vi "format file size and count.vi"(11 "size":i64) -> (3 "size":string)   [LabVIEW 2023]
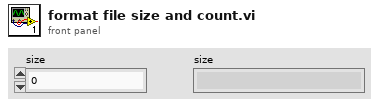
[diagram p1: front panel]
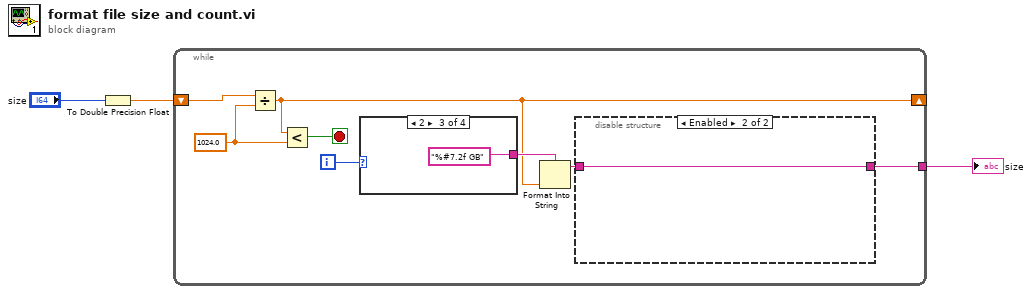
[diagram p0: block diagram]
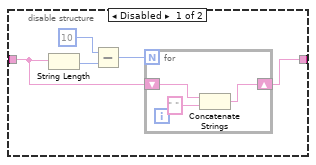
[diagram p2: hidden frame]
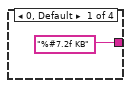
[diagram p3: hidden frame]
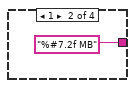
[diagram p4: hidden frame]
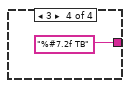
[diagram p5: hidden frame]
diagram:
  n1 = To Double Precision Float(number="size") -> (double precision float=w2:dbl)
  n2 = while {
    shift-right: [w6] -> _
    shift-left: w2 -> [w8]
    tunnel: [w4] -> w1
    i -> [w9]
    stop <- w10 stop-if-true
    w11 = 1024.0 ("y")
    n3 = Divide(x=w8, y=w11) -> (x/y=w6:dbl)
    n4 = Less?(x=w6, y=w11) -> (x < y?=w10:bool)
    n5 = case shown="2" w9 {
      tunnel: ["%#7.2f KB" ("String 2") "%#7.2f MB" ("String 2") "%#7.2f GB" ("String 2") "%#7.2f TB" ("String 2")] -> w7
      frame 0, Default {
      }
      frame 1 {
      }
      frame 2 {
      }
      frame 3 {
      }
    }
    n6 = Format Into String(format string=w7, w6) -> (resulting string=w5:string)  [unwired: 2 in, 1 out]
    n7 = disable-structure shown="Enabled" {
      disable-tunnel: w5 -> [w13 w20]
      disable-tunnel: [w12 w20] -> w4
      frame Disabled {
        n8 = String Length(string=w13) -> (length=w16:i32)
        n9 = Subtract(x=10, y=w16) -> (x-y=w15:i32)
        n10 = for {
          N: w15 -> [_]
          shift-right: [w18] -> w12
          shift-left: w13 -> [w19]
          n11 = Concatenate Strings(w19, " " ("string")) -> (w18:string)
        }
      }
      frame Enabled {
      }
    }
  }
  "size" <- w1
